vi "Sensor Refname to String.vi"(1 "Sensor Refnames":T1) -> (0 "Refname":string)   [LabVIEW 2014]
uses:
  Sensor Refname.ctl
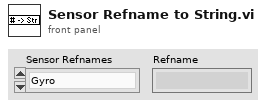
[diagram p1: front panel]
types:
  T1 = typedef "Sensor Refname.ctl" = enum16{"Gyro", "Elevator Top LS", "Elevator Bottom LS", "Claw Outside LS", "Left Drive Encoder", "Right Drive Encoder", "Strafe Encoder", "Elevator Encoder", "Ultrasonic Forward", "Ultrasonic Back", "Arm Angle POT", "Arm Clapper POT", "Accelerometer", "Tote LS", "DIP 1", "DIP 2", "DIP 3", "DIP 4"}
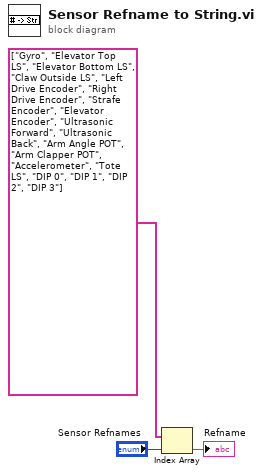
[diagram p0: block diagram]
diagram:
  n1 = Index Array(array=string[] ["Gyro", "Elevator Top LS", "Elevator Bottom LS", "Claw Outside LS", "Left Drive Encoder", "Right Drive Encoder", "Strafe Encoder", "Elevator Encoder", "Ultrasonic Forward", "Ultrasonic Back", "Arm Angle POT", "Arm Clapper POT", "Accelerometer", "Tote LS", "DIP 0", "DIP 1", "DIP 2", "DIP 3"] ("Strings []"), index="Sensor Refnames") -> (element=→"Refname":string)
